vi "ReadFromFIFOPort3.vi"(10 "stop":bool) -> (2 "This is what I told you!":string)   [LabVIEW 2011]
doc: "Elizabeth Mahon\nBased off of example from LabView and IGVC 3.2.1 Read VectorNav.\nReads data from compass sensor on port 1 of the serial module from a FIFO and outputs it as a string.\nStarts as waiting, then when it reads $ (first element of compass string) starts reading and adds everything it reads together until it reaches *ss (where ss can be anything, the \"two digit checksum\"), and then stops and outputs the string.\nOnly reads the string once - must be run in a while loop for multiple readings.\nJust shuts down if it has an error. In the future, we might want to output if it has an error."
uses:
  <vilib>/rvi/interface/nirviOpenFPGA/nirviOpenFPGA.xnode
  <vilib>/rvi/interface/nirviMethod/nirviMethod.xnode
  <vilib>/FPGAPlugInAG/Dynamic/niLvFpga_ReadFifo_Dynamic.vi
  <vilib>/rvi/errors/niLvFpgaMergeErrorWithErrorCode.vi
  <vilib>/rvi/interface/nirviCloseFPGA/nirviCloseFPGA.xnode
  <vilib>/FPGAPlugInAG/Dynamic/niLvFpga_Close_Dynamic.vi
  1A-FPGA/1A Code/WriteToFIFOPort3.vi
panel:
  out "Current Status":enum16{"Waiting", "Reading", "Time Out!"}(ring)
  out "Data":i16[](array[numeric])
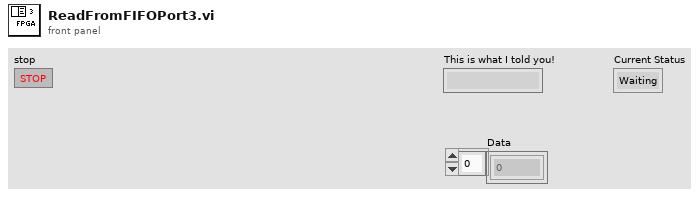
[diagram p1: front panel]
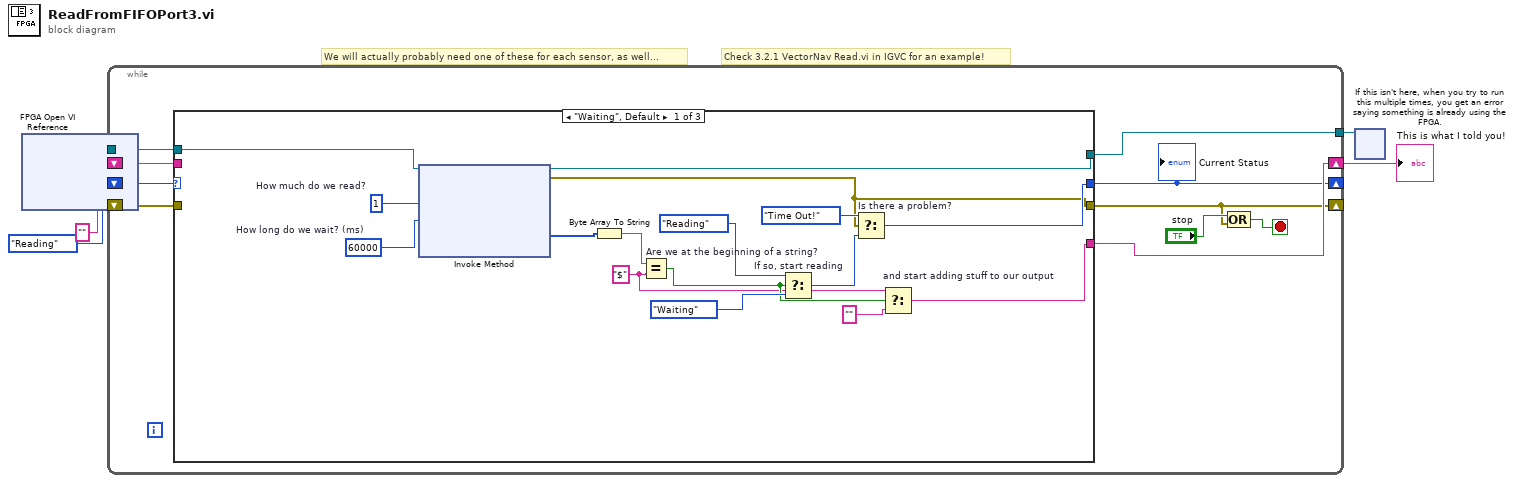
[diagram p0: block diagram]
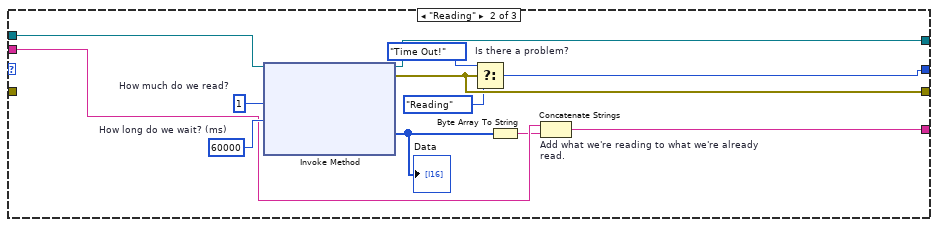
[diagram p2: hidden frame]
diagram:
  # "Check 3.2.1 VectorNav Read.vi in IGVC for an example!"
  # "We will actually probably need one of these for each sensor, as well..."
  n1 = xnode "FPGA Open VI Reference"() -> ("FPGA VI Reference Out"=w5:refnum<k20>)  [unwired: 2 in, 1 out]
  n2 = while {
    tunnel: w5 -> [w15]
    shift-right: [w13] -> w4
    shift-left: "" -> [w14]
    shift-right: [w6] -> _
    shift-left: enum16{"Waiting", "Reading", "Time Out!"}."Reading" ("Status") -> [w12]
    shift-right: [w9] -> _
    shift-left: _ -> [w8]
    tunnel: [w7] -> w1
    stop <- w10 stop-if-true
    n3 = case shown="\"Waiting\", Default" w12 {
      selector: w12 -> [_ _ w47]
      tunnel: w15 -> [w31 w41 w44]
      tunnel: w14 -> [_ w36 w46]
      tunnel: [w18 w37 w46] -> w13
      tunnel: [w22 w39 w47] -> w6
      tunnel: [w21 w38 w45] -> w9
      tunnel: w8 -> [_ _ w45]
      tunnel: [w30 w34 w44] -> w7
      frame "Waiting", Default {
        w17 = "$" ("x")
        w28 = 60000  # How long do we wait? (ms)
        w29 = u32 1  # How much do we read?
        n4 = xnode "Invoke Method"("FPGA VI Reference In"=w31, "Number of Elements"=w29, "Timeout (ms)"=w28) -> ("FPGA VI Reference Out"=w30:refnum<k20>, "error out"=w21:errorcluster, "Data"=w27:u8[])  [unwired: 1 in, 1 out]
        n5 = Byte Array To String(unsigned byte array=w27) -> (string=w16:string)
        n6 = Equal? "Are we at the beginning of a string?"(x=w16, y=w17) -> (x = y?=w19:bool)
        n7 = Select "If so, start reading"(t=enum16{"Waiting", "Reading", "Time Out!"}."Reading", s=w19, f=enum16{"Waiting", "Reading", "Time Out!"}."Waiting" ("Current Status")) -> (s? t:f=w24:enum16{"Waiting", "Reading", "Time Out!"})
        n8 = Select "Is there a problem?"(t=enum16{"Waiting", "Reading", "Time Out!"}."Time Out!", s=w21, f=w24) -> (s? t:f=w22:enum16{"Waiting", "Reading", "Time Out!"})
        n9 = Select "and start adding stuff to our output"(t=w17, s=w19, f="") -> (s? t:f=w18:string)
      }
      frame "Reading" {
        w42 = 60000  # How long do we wait? (ms)
        w43 = u32 1  # How much do we read?
        n10 = xnode "Invoke Method"("FPGA VI Reference In"=w41, "Number of Elements"=w43, "Timeout (ms)"=w42) -> ("FPGA VI Reference Out"=w34:refnum<k20>, "error out"=w38:errorcluster, "Data"=w40:u8[])  [unwired: 1 in, 1 out]
        "Data" <- w40
        n11 = Select "Is there a problem?"(t=enum16{"Waiting", "Reading", "Time Out!"}."Time Out!", s=w38, f=enum16{"Waiting", "Reading", "Time Out!"}."Reading" ("Status")) -> (s? t:f=w39:enum16{"Waiting", "Reading", "Time Out!"})
        n12 = Byte Array To String(unsigned byte array=w40) -> (string=w35:string)
        n13 = Concatenate Strings "Add what we're reading to what we're already read."(w36, w35) -> (w37:string)
      }
      frame "Time Out!" {
        # "error or something. Not sure what to do."
      }
    }
    "Current Status" <- w6
    n14 = Compound Arithmetic op=OR("stop", w9) -> (w10:bool)
  }
  "This is what I told you!" <- w4
  n15 = xnode "If this isn't here, when you try to run\nthis multiple times, you get an error\nsaying something is already using the\nFPGA."("FPGA VI Reference In"=w1) -> ()  [unwired: 1 in, 1 out]
